vi "StatMon_AH2700.vi"(7 "System Monitor Variables":T1, 9 "Scale Meas Op":dbl=1.0, 11 "Update AH":bool) -> (0 "Meas Op Y":string, 1 "Meas Op X":string, 2 "Out 2":dbl[](array[numeric]), 3 "Out 1":dbl[](array[numeric]), 4 "Meas Op Z":string, 5 "Scaled":dbl[][](array[numeric]))   [LabVIEW 2019]
uses:
  Global/Global Variables/System Monitor Cluster.ctl
  Global/Global Variables/Data_Display_global.vi
panel:
  in  "Meas Op Ch 2":bool
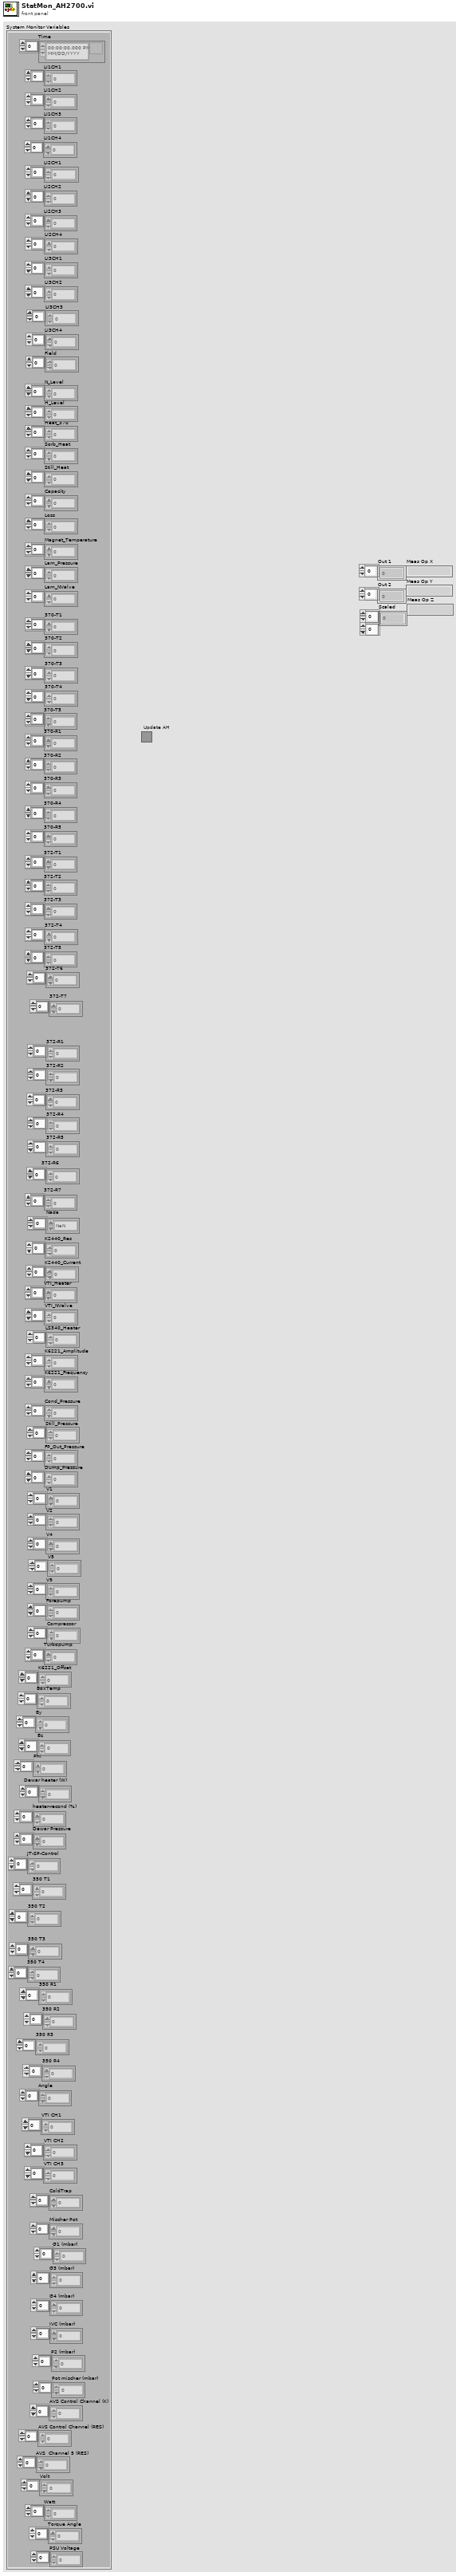
[diagram p1: front panel]
types:
  T1 = typedef "System Monitor Cluster.ctl" = cluster{"Time":timestamp[], "LI1CH1":dbl[], "LI1CH2":dbl[], "LI2CH1":dbl[], "LI2CH2":dbl[], "LI3CH1":dbl[], "LI3CH2":dbl[], "Field":dbl[], "N_Level":dbl[], "H_Level":dbl[], "Heat_370":dbl[], "Sorb_Heat":dbl[], "Still_Heat":dbl[], "Capacity":dbl[], "Loss":dbl[], "Magnet_Temperature":dbl[], "Lam_Pressure":dbl[], "Lam_NValve":dbl[], "370-T1":dbl[], "370-T2":dbl[], "370-T3":dbl[], "370-T4":dbl[], "370-T5":dbl[], "370-R1":dbl[], "370-R2":dbl[], "370-R3":dbl[], "370-R4":dbl[], "370-R5":dbl[], "372-T1":dbl[], "372-T2":dbl[], "372-T3":dbl[], "372-T4":dbl[], "372-T5":dbl[], "372-T6":dbl[], "372-R1":dbl[], "372-R2":dbl[], "372-R3":dbl[], "372-R4":dbl[], "372-R5":dbl[], "372-R6":dbl[], "Nada":dbl[], "K2440_Res":dbl[], "K2440_Current":dbl[], "VTI_Heater":dbl[], "VTI_NValve":dbl[], "LS340_Heater":dbl[], "K6221_Amplitude":dbl[], "K6221_Frequency":dbl[], "Cond_Pressure":dbl[], "Still_Pressure":dbl[], "FP_Out_Pressure":dbl[], "Dump_Pressure":dbl[], "V1":dbl[], "V2":dbl[], "V4":dbl[], "V5":dbl[], "V9":dbl[], "Forepump":dbl[], "Compressor":dbl[], "K6221_Offset":dbl[], "BoxTemp":dbl[], "By":dbl[], "Bz":dbl[], "Phi":dbl[], "heater-recond (%)":dbl[], "Dewar Pressure ":dbl[], "JT-SP-Control":dbl[], "350 T1":dbl[], "350 T2":dbl[], "350 T3":dbl[], "350 T4":dbl[], "350 R1":dbl[], "350 R2":dbl[], "350 R3":dbl[], "350 R4":dbl[], "Angle":dbl[], "VTI CH1":dbl[], "VTI CH2":dbl[], "VTI CH3":dbl[], "ColdTrap":dbl[], "Mischer Pot":dbl[], "G1 (mbar)":dbl[], "G3 (mbar) ":dbl[], "G4 (mbar)":dbl[], "IVC (mbar)":dbl[], "P2 (mbar) ":dbl[], "Pot mischer (mbar)":dbl[], "AVS Control Channel (K)":dbl[], "AVS Control Channel (RES)":dbl[], "AVS  Channel 5 (RES) ":dbl[], "LI3CH3":dbl[], "LI3CH4":dbl[], "LI1CH3":dbl[], "LI1CH4":dbl[], "LI2CH3":dbl[], "LI2CH4":dbl[], "Volt":dbl[], "Watt":dbl[], "Torque Angle":dbl[], "Dewar heater (W)":dbl[], "PSU Voltage":dbl[], "Turbopump":dbl[], "372-R7":dbl[], "372-T7":dbl[]}
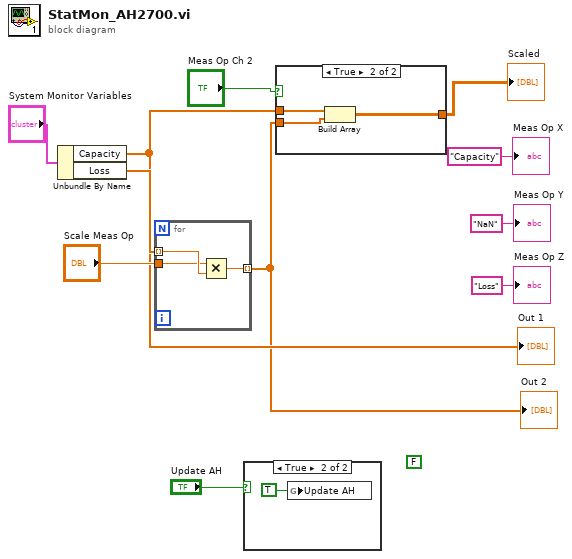
[diagram p0: block diagram]
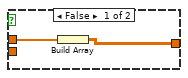
[diagram p2: hidden frame]
diagram:
  (unwired) FALSE
  n1 = Unbundle By Name("System Monitor Variables") -> ("Capacity"=w6:dbl[], "Loss"=w10:dbl[])
  "Out 1" <- w6
  n2 = for {
    tunnel: w10 -> [w14] mode=indexing
    tunnel: "Scale Meas Op" -> [w13]
    tunnel: [w12] -> w5 mode=indexing
    n3 = Multiply(x=w13, y=w14) -> (x*y=w12:dbl)
  }
  "Out 2" <- w5
  n4 = case shown="True" "Update AH" {
    frame False {
    }
    frame True {
      n5 = global write "Data_Display_global.vi" "Update AH"(TRUE) -> ()
    }
  }
  n6 = case shown="True" "Meas Op Ch 2" {
    tunnel: w6 -> [w17 w20]
    tunnel: [w16 w19] -> w1
    tunnel: w5 -> [_ w18]
    frame False {
      n7 = Build Array(w17) -> (w16:dbl[][])
    }
    frame True {
      n8 = Build Array(w20, w18) -> (w19:dbl[][])
    }
  }
  "Scaled" <- w1
  "Meas Op X" <- "Capacity"
  "Meas Op Y" <- "NaN"
  "Meas Op Z" <- "Loss"
